vi "Readename.vi"(8 "error in (no error)":errorcluster, 11 "object in":refnum<class "error Message.lvclass">) -> (0 "error out":errorcluster, 2 "ename":string, 3 "object out":refnum<class "error Message.lvclass">)   [LabVIEW 2018, in "ClientMessaging.lvlib" / "error Message.lvclass"]
uses:
  error Message.lvclass
  error Message.lvclass/error Message.ctl
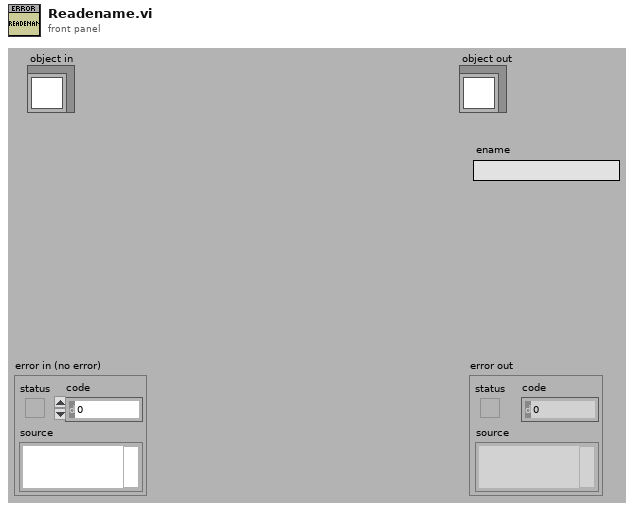
[diagram p1: front panel]
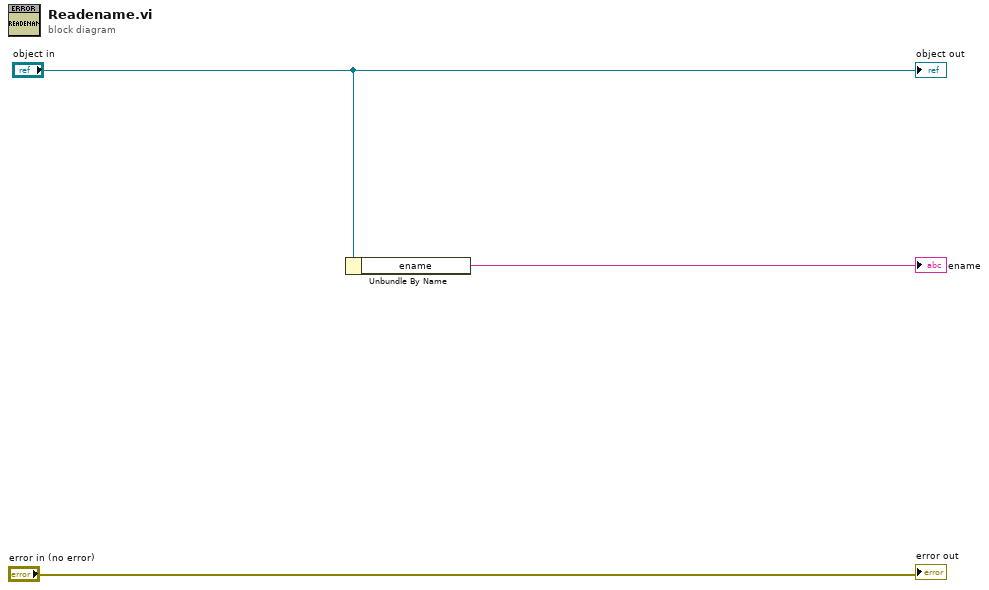
[diagram p0: block diagram]
diagram:
  n1 = Unbundle By Name("object in") -> ("ename"=→"ename":string)
  "error out" <- "error in (no error)"
  "object out" <- "object in"
